vi "Text Description.vi"(11 "Relabel in":refnum<class "Relabel.lvclass">) -> (2 "Description":string, 3 "Relabel out":refnum<class "Relabel.lvclass">)   [LabVIEW 2011, in "Messenging.lvlib" / "Relabel.lvclass"]
uses:
  Relabel.lvclass
  Relabel.lvclass/Relabel.ctl
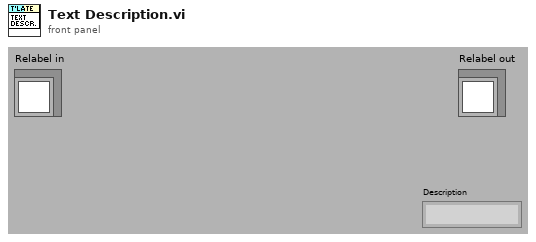
[diagram p1: front panel]
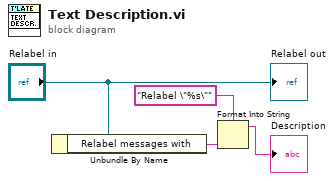
[diagram p0: block diagram]
diagram:
  n1 = Unbundle By Name("Relabel in") -> ("Relabel messages with"=w2:string)
  n2 = Format Into String(format string="Relabel \"%s\"", w2) -> (resulting string=→"Description":string)  [unwired: 2 in, 1 out]
  "Relabel out" <- "Relabel in"
